vi "IMAQ FPGA Camera Link 1 Tap 12-Bit.vi"(6 "Ready for Output":bool=TRUE, 7 "Camera Link Enables":T2, 8 "Cancel Acquisition":bool, 9 "Acquire":bool=TRUE, 10 "Camera Link Data":cluster{"Port A":u8, "Port B":u8}, 11 "Acquisition Settings":T3) -> (0 "Output Valid":bool, 2 "Acquisition Status":T1, 3 "Vision Pixel Bus Out":T4, 5 "Acquisition Overflow":bool)   [LabVIEW 2017]
doc: "Acquires images from a 1 tap 12-bit (1X1-1Y) Camera Link Camera. On each pixel clock, a single pixel arrives starting at the left of the image. Ensure that this VI is called from a Single Cycle Timed Loop that is running faster than the pixel clock of the camera.\n\nThe <B>Vision Pixel Bus Out</B> can be connected to Vision FPGA algorithms for processing."
uses:
  <vilib>/visionFPGA/Controls/IMAQ FPGA Pixel Bus u16x1.ctl
  <vilib>/visionFPGA/Basics/Camera Link Acquisition/CL Data to Pixels/IMAQ FPGA Camera Link Data to Pixels 1 Tap 12-Bit.vi
  <vilib>/visionFPGA/Basics/Camera Link Acquisition/Pixel Bus to Vision Pixel Bus/IMAQ FPGA Camera Link Pixel Bus to Vision Pixel Bus U16x1.vi
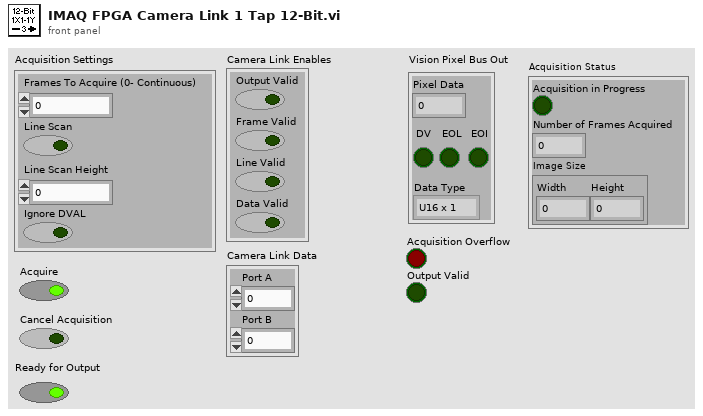
[diagram p1: front panel]
types:
  T1 = cluster{"Acquisition in Progress":bool, "Number of Frames Acquired":u32, "Image Size":cluster{"Width":u32, "Height":u32}}
  T2 = cluster{"Output Valid":bool, "Frame Valid":bool, "Line Valid":bool, "Data Valid":bool}
  T3 = cluster{"Frames To Acquire (0- Continuous)":u32, "Line Scan":bool, "Line Scan Height":u32, "Ignore DVAL":bool}
  T4 = typedef "IMAQ FPGA Pixel Bus u16x1.ctl" = cluster{"Pixel Data":u16, "DV":bool, "EOL":bool, "EOI":bool, "Data Type":enum16{"U16 x 1"}}
  T5 = cluster{"Acquisition in Progress":bool, "Num Frames Acquired":u32, "Height":u32, "Number of Cycles per Line":u32}
  T6 = cluster{"Number of Cycles per Line":u32, "Height":u32}
  T7 = cluster{"Acquisition in Progress":bool, "Num Frames Acquired":u32, cluster{"Number of Cycles per Line":u32, "Height":u32}}
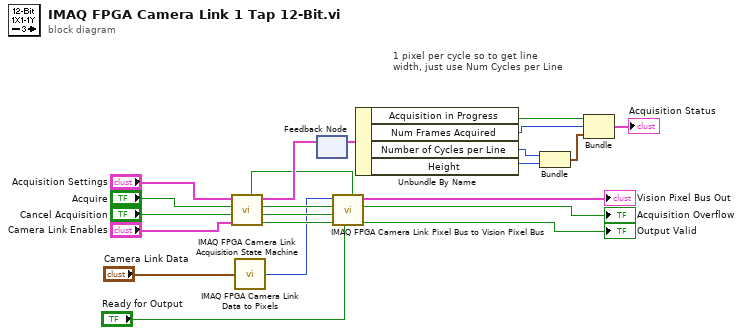
[diagram p0: block diagram]
diagram:
  # "1 pixel per cycle so to get line width, just use Num Cycles per Line"
  n1 = call <vilib>:"IMAQ FPGA Camera Link Acquisition State Machine.vi"("Enables"="Camera Link Enables", "Cancel Acq"="Cancel Acquisition", "Acquire"="Acquire", "Acquisition Settings"="Acquisition Settings") -> ("Output Valid"=w13:bool, "Frame Valid"=w14:bool, "Line Valid"=w15:bool, "Acquisition Status"=w17:T5, "Reset"=w5:bool)  [unwired: 3 in]
  n2 = call-poly <vilib>:"IMAQ FPGA Camera Link Data to Pixels.vi"("Camera Link Data"="Camera Link Data") -> ("Pixel"=w6:u16)
  n3 = feedback #1() -> (w8:T5)  [unwired: 1 in]
  n4 = feedback-in #1(w17) -> ()
  n5 = call-poly <vilib>:"IMAQ FPGA Camera Link Pixel Bus to Vision Pixel Bus.vi"("Reset Overflow"=w5, "Ready for Output"="Ready for Output", "Input Valid"=w13, "Frame Valid In"=w14, "Line Valid In"=w15, "Pixel In"=w6) -> ("Output Valid"=→"Output Valid":bool, "Acquisition Overflow"=→"Acquisition Overflow":bool, "Vision Pixel Bus Out"=→"Vision Pixel Bus Out":T4)  [unwired: 3 in]
  n6 = Unbundle By Name(w8) -> ("Acquisition in Progress"=w4:bool, "Num Frames Acquired"=w3:u32, "Number of Cycles per Line"=w16:u32, "Height"=w22:u32)
  n7 = Bundle("Number of Cycles per Line"=w16, "Height"=w22) -> (w2:T6)  [unwired: 1 in]
  n8 = Bundle("Acquisition in Progress"=w4, "Num Frames Acquired"=w3, w2) -> (→"Acquisition Status":T7)  [unwired: 1 in]
